vi "LSMcontroller_v66_improvedwfhandling.vi"() -> ()   [LabVIEW 2015] (continued)
                            n1708 = case shown="False" w4683 {
                              frame False {
                                n1709 = disable-structure shown="Disabled" {
                                frame Disabled {
                                n1710 = call "2pparameters.vi"("command"="get") -> ("params out"=w4685:T10)  [unwired: 1 in]
                                n1711 = Unbundle By Name(w4685) -> ("autoshutter"=w4686:bool)
                                n1712 = case shown="True" w4686 {
                                frame False {
                                }
                                frame True {
                                n1713 = call "shuttercontrol.vi"("command"="open") -> ()  [unwired: 1 in, 1 out]
                                }
                                }
                                }
                                frame Enabled {
                                }
                                }
                              }
                              frame True {
                              }
                            }
                          }
                          frame #4 {
                            n1714 = flat-sequence {
                              frame #0 {
                                # "Disabled for conversion to 64 bit"
                                n1715 = disable-structure shown="Disabled" {
                                frame Disabled {
                                n1716 = local read "Measurement"() -> (w4689:T4)
                                n1717 = case shown="\"Lifetime (contour)\"" w4689 {
                                frame "X-Y-t movie", Default {
                                }
                                frame "Lifetime (contour)" {
                                n1718 = call "runLT_img.vi"() -> ()  [unwired: 1 in]
                                }
                                }
                                }
                                frame Enabled {
                                }
                                }
                                n1719 = local write "64bit disabled"(TRUE ("64bit disabled")) -> ()
                              }
                              frame #1 {
                                n1720 = call "runAI_img.vi"() -> ()  [unwired: 12 in]
                                n1721 = call "runCI.vi"() -> ()  [unwired: 12 in]
                                n1722 = call "runDO_img.vi"() -> ()  [unwired: 12 in]
                              }
                              frame #2 {
                                n1723 = call "runAO_img.vi"() -> ()  [unwired: 12 in]
                              }
                            }
                          }
                          frame #5 {
                            # "Disabled for conversion to 64 bit"
                            n1724 = disable-structure shown="Disabled" {
                              disable-tunnel: w4691 -> [w4692 _]
                              frame Disabled {
                                w4695 = u16 0 items=["Stream to disk", "Post process", "real time process"] ("Ring")
                                n1725 = local read "T3R Data processing"() -> (w4694:u16)
                                n1726 = Equal?(x=w4694, y=w4695) -> (x = y?=w4693:bool)
                                n1727 = local read "save\ndata"() -> (w4697:bool)
                                n1728 = local read "Measurement"() -> (w4698:T4)
                                n1729 = And(x=w4697, y=w4693) -> (x .and. y?=w4696:bool)
                                n1730 = case shown="\"Lifetime (contour)\"" w4698 {
                                tunnel: w4692 -> [_ w4702]
                                tunnel: w4696 -> [_ w4700]
                                frame "X-Y-t movie", Default {
                                }
                                frame "Lifetime (contour)" {
                                n1731 = case shown="True" w4700 {
                                selector: w4700 -> [w4703 w4708]
                                tunnel: w4702 -> [_ w4706]
                                tunnel: [path "" ("appended path") w4709] -> w4701
                                tunnel: [w4703 w4708] -> w4699
                                frame False {
                                }
                                frame True {
                                n1732 = local read "filename prefix"() -> (w4707:string)
                                n1733 = local read "data dir"() -> (w4710:path)
                                n1734 = call "generatedatafilename.vi"("timestamp"=w4706, "filename prefix in"=w4707) -> ("full-filename"=w4705:string)
                                n1735 = Concatenate Strings(w4705, ".lvpt3contour" ("string")) -> (w4712:string)
                                n1736 = Build Path(base path=w4710, name or relative path=w4712) -> (appended path=w4709:path)
                                }
                                }
                                n1737 = call "collectLT_res_v1.vi"("stream?"=w4699, "data file"=w4701) -> ()  [unwired: 2 out]
                                }
                                }
                              }
                              frame Enabled {
                              }
                            }
                            n1738 = while {
                              i -> [w4715]
                              stop <- w4713 stop-if-true
                              n1739 = local read "Stop"() -> (w4723:bool)
                              n1740 = local read "Exit"() -> (w4722:bool)
                              n1741 = Increment(x=w4715) -> (x+1=w4714:i32)
                              n1742 = local write "points recorded"(w4714) -> ()
                              n1743 = Or(x=w4723, y=w4722) -> (x .or. y?=w4721:bool)
                              n1744 = case shown="False" w4721 {
                                frame False {
                                n1745 = stacked-sequence {
                                frame #0 {
                                n1746 = call "collectAI_tt_V2.vi"() -> ()  [unwired: 4 in]
                                n1747 = call "collectCI_tt.vi"() -> ("size(s)"=w4730:i32)  [unwired: 3 in]
                                n1748 = local write "scol"(w4730) -> ()
                                }
                                frame #1 {
                                n1749 = local read "Live"() -> (w4731:bool)
                                n1750 = case shown="True" w4731 {
                                frame False {
                                }
                                frame True {
                                n1751 = local read "graph1list"() -> (w4738:u16)
                                n1752 = local read "graph2list"() -> (w4737:u16)
                                n1753 = To Unsigned Word Integer(number=w4738) -> (unsigned 16bit integer=w4736:u16)
                                n1754 = To Unsigned Word Integer(number=w4737) -> (unsigned 16bit integer=w4735:u16)
                                n1755 = call "dattotrace.vi"("graph2list"=w4735, "Current Average"=sgl 1.0, "graph1list"=w4736) -> ("trace2array out"=w4733:sgl[], "trace1array out"=w4744:sgl[])
                                n1756 = local read "bin"() -> (w4745:dbl)
                                n1757 = script code="data=reshape(datain,[bin length(datain)./bin]);\ndataout=mean(data,1);\ndata2=reshape(datain2,[bin length(datain2)./bin]);\ndataout2=mean(data2,1);"("bin"=w4745, "datain"=w4744, "datain2"=w4733) -> ("dataout"=w4743:dbl[], "dataout2"=w4732:dbl[])  [unwired: 1 in, 1 out]
                                n1758 = Array Size(array=w4732) -> (size(s)=w4746:i32)
                                n1759 = Divide(x=w4746, y=2) -> (x/y=w4748:dbl)
                                n1760 = Round To Nearest(number=w4748) -> (nearest integer value=w4750:dbl)
                                n1761 = Array Size(array=w4743) -> (size(s)=w4755:i32)
                                n1762 = Delete From Array(array=w4732, length=w4750, index=0) -> (deleted portion=w4741:dbl[], array with subset deleted=w4742:dbl[])
                                n1763 = Divide(x=w4755, y=2) -> (x/y=w4753:dbl)
                                n1764 = Round To Nearest(number=w4753) -> (nearest integer value=w4751:dbl)
                                n1765 = Delete From Array(array=w4743, length=w4751, index=0) -> (deleted portion=w4740:dbl[], array with subset deleted=w4739:dbl[])
                                n1766 = local write "graph2"(w4739) -> ()
                                n1767 = local write "graph1"(w4740) -> ()
                                n1768 = local write "graph3"(w4741) -> ()
                                n1769 = local write "graph4"(w4742) -> ()
                                }
                                }
                                }
                                frame #2 {
                                n1770 = local read "save\ndata"() -> (w4756:bool)
                                n1771 = case shown="True" w4756 {
                                frame False {
                                }
                                frame True {
                                n1772 = call "savebinaryfiles.vi"() -> ()  [unwired: 1 in]
                                }
                                }
                                }
                                }
                                }
                                frame True {
                                }
                              }
                              n1773 = local read "continuous"() -> (w4718:bool)
                              n1774 = case shown="False" w4718 {
                                tunnel: w4714 -> [w4728 _]
                                tunnel: [w4727 FALSE] -> w4716
                                frame False {
                                n1775 = call "2pparameters.vi"("command"="get") -> ("params out"=w4725:T10)  [unwired: 1 in]
                                n1776 = Unbundle By Name(w4725) -> ("tt_cycles"=w4724:i32)
                                n1777 = Greater Or Equal?(x=w4728, y=w4724) -> (x >= y?=w4727:bool)
                                }
                                frame True {
                                }
                              }
                              n1778 = local read "Stop"() -> (w4720:bool)
                              n1779 = local read "Exit"() -> (w4719:bool)
                              n1780 = Or(x=w4720, y=w4719) -> (x .or. y?=w4717:bool)
                              n1781 = Or(x=w4717, y=w4716) -> (x .or. y?=w4713:bool)
                            }
                            n1782 = local write "64bit disabled"(TRUE ("64bit disabled")) -> ()
                          }
                          frame #6 {
                            # "Disabled for conversion to 64 bit"
                            n1783 = local read "Measurement"() -> (w4759:T4)
                            n1784 = disable-structure shown="Disabled" {
                              disable-tunnel: w4759 -> [w4761 _]
                              disable-tunnel: w4758 -> [w4760 _]
                              frame Disabled {
                                n1785 = case shown="\"Lifetime (contour)\"" w4761 {
                                tunnel: w4760 -> [_ w4762]
                                frame "X-Y-t movie", Default {
                                }
                                frame "Lifetime (contour)" {
                                n1786 = stacked-sequence {
                                tunnel: w4762 -> [_ w4763]
                                frame #0 {
                                n1787 = flat-sequence {
                                frame #0 {
                                n1788 = call "stoperaseLT_img.vi"() -> ()  [unwired: 1 in]
                                }
                                }
                                }
                                frame #1 {
                                w4766 = u16 0 items=["Stream to disk", "Post process", "real time process"] ("Ring")
                                n1789 = local read "T3R Data processing"() -> (w4765:u16)
                                n1790 = local read "save\ndata"() -> (w4768:bool)
                                n1791 = Equal?(x=w4765, y=w4766) -> (x = y?=w4764:bool)
                                n1792 = Not(x=w4764) -> (.not. x?=w4769:bool)
                                n1793 = And(x=w4768, y=w4769) -> (x .and. y?=w4767:bool)
                                n1794 = case shown="True" w4767 {
                                tunnel: w4763 -> [_ w4770]
                                frame False {
                                }
                                frame True {
                                n1795 = local read "filename prefix"() -> (w4771:string)
                                n1796 = local read "data dir"() -> (w4787:path)
                                n1797 = call "2pparameters.vi"("command"="get") -> ("params out"=w4782:T10)  [unwired: 1 in]
                                n1798 = call "generatedatafilename.vi"("timestamp"=w4770, "filename prefix in"=w4771) -> ("full-filename"=w4772:string)
                                n1799 = Unbundle By Name(w4782) -> ("srate"=w4780:sgl, "Pel"=w4779:sgl, "measpoints"=w4777:i32)
                                n1800 = Concatenate Strings(w4772, ".lvpt3contour" ("string")) -> (w4785:string)
                                n1801 = Build Path(base path=w4787, name or relative path=w4785) -> (appended path=w4784:path)
                                n1802 = To Unsigned Long Integer(number=w4780) -> (unsigned 32bit integer=w4781:u32)
                                n1803 = To Unsigned Long Integer(number=w4779) -> (unsigned 32bit integer=w4778:u32)
                                n1804 = To Unsigned Long Integer(number=w4777) -> (unsigned 32bit integer=w4776:u32)
                                n1805 = call "PH-temp-raw.vi"("command"="get") -> ("array out"=w4775:u32[])  [unwired: 1 in]
                                n1806 = Build Array (concatenate)(w4781, w4778, w4776, w4775) -> (w4774:u32[])
                                n1807 = Open/Create/Replace File(file path (use dialog)=w4784, operation (0:open)=T8."replace or create") -> (refnum out=w4791:refnum<file>, error out=w4790:errorcluster)  [unwired: 4 in, 1 out]
                                n1808 = Write to Binary File(file (use dialog)=w4791, data=w4774, error in=w4790, 5:FALSE ("prepend array or string size? (T)")) -> (refnum out=w4788:refnum<file>, error out=w4789:errorcluster)  [unwired: 2 in, 1 out]
                                n1809 = Close File(refnum=w4788, error in=w4789) -> ()  [unwired: 2 out]
                                }
                                }
                                }
                                }
                                }
                                }
                              }
                              frame Enabled {
                              }
                            }
                            n1810 = local write "64bit disabled"(TRUE ("64bit disabled")) -> ()
                          }
                          frame #7 {
                            n1811 = call "reset AO_DO_v3.vi"() -> ()  [unwired: 12 in]
                          }
                          frame #8 {
                            n1812 = stacked-sequence {
                              tunnel: w4807 -> [w4810 _ _ _ _ _]
                              tunnel: w4804 -> [w4809 _ _ _ _ _]
                              tunnel: w4805 -> [w4808 _ _ _ _ _]
                              tunnel: w4806 -> [_ w4859 _ _ _ _]
                              tunnel: w4802 -> [_ w4858 w4913 w5010 _ _]
                              tunnel: w4803 -> [_ w4857 w4912 w5009 _ _]
                              tunnel: w4801 -> [_ _ _ w5008 _ _]
                              tunnel: w4800 -> [_ _ _ w5007 _ _]
                              tunnel: w4799 -> [_ _ w4910 _ _ _]
                              tunnel: w4798 -> [_ _ w4909 _ _ _]
                              tunnel: w4797 -> [_ _ w4907 _ _ _]
                              tunnel: w4796 -> [_ _ w4906 _ _ _]
                              tunnel: w4795 -> [_ _ _ w5005 _ _]
                              tunnel: w4794 -> [_ _ _ w5004 _ _]
                              frame #0 {
                                n1813 = case shown="False" w4810 {
                                tunnel: w4809 -> [_ w4832]
                                tunnel: w4808 -> [_ w4831]
                                frame True {
                                n1814 = stacked-sequence {
                                seq-local: [w4811 _ _] -> [_ w4823 w4828]
                                frame #0 {
                                n1815 = call "configuration.vi"("command"="get") -> ("config out"=w4817:T11)  [unwired: 2 in, 1 out]
                                n1816 = Unbundle By Name(w4817) -> ("Voltage to Xgalvo"=w4814:i32)
                                n1817 = call "2pparameters.vi"("command"="get") -> ("params out"=w4815:T10)  [unwired: 1 in]
                                n1818 = in-place {
                                in-place-border: w4814 -> [w4822]
                                in-place-border: [w4819] -> w4811
                                n1819 = in-place-cluster #31(w4815) -> ("aAO"=w4821:u32[])
                                n1820 = call "remove channel from active arrayv2.vi"("line array in"=w4821, "line to remove"=w4822) -> ("line array out"=w4820:u32[], "index"=w4819:i32)  [unwired: 1 out]
                                n1821 = in-place-cluster #31("aAO"=w4820) -> (w4812:T10)
                                }
                                n1822 = call "2pparameters.vi"("Params in"=w4812, "command"="set") -> ()  [unwired: 1 out]
                                }
                                frame #1 {
                                n1823 = call "waveformparamsv2.vi"("command"="rem AO", "index"=w4823) -> ()  [unwired: 3 in, 3 out]
                                }
                                frame #2 {
                                n1824 = call "waveformsAObuffer.vi"("command"="get") -> ("AO wf out"=w4829:waveform(dbl)[])  [unwired: 1 in]
                                n1825 = Delete From Array(array=w4829, length=1, index=w4828) -> (array with subset deleted=w4825:waveform(dbl)[])  [unwired: 1 out]
                                n1826 = call "waveformsAObuffer.vi"("AO wf in"=w4825, "command"="set") -> ()  [unwired: 1 out]
                                }
                                }
                                }
                                frame False {
                                n1827 = stacked-sequence {
                                seq-local: [w4833 _ _] -> [_ w4841 w4852]
                                tunnel: w4832 -> [_ w4840 _]
                                tunnel: w4831 -> [_ _ w4851]
                                frame #0 {
                                n1828 = call "configuration.vi"("command"="get") -> ("config out"=w4838:T11)  [unwired: 2 in, 1 out]
                                n1829 = Unbundle By Name(w4838) -> ("Voltage to Xgalvo"=w4834:i32)
                                n1830 = call "2pparameters.vi"("command"="get") -> ("params out"=w4837:T10)  [unwired: 1 in]
                                n1831 = Unbundle By Name(w4837) -> ("aAO"=w4835:u32[])
                                n1832 = Search 1D Array(1D array=w4835, element=w4834) -> (index of element=w4833:i32)  [unwired: 1 in]
                                }
                                frame #1 {
                                n1833 = call "waveformparamsv2.vi"("command"="get") -> ("Params out"=w4844:T14)  [unwired: 4 in, 2 out]
                                n1834 = in-place {
                                in-place-border: w4841 -> [w4848]
                                in-place-border: w4840 -> [w4847]
                                n1835 = in-place-cluster #32(w4844) -> ("AO parameters"=w4849:T15)
                                n1836 = in-place {
                                in-place-border: w4847 -> [w4850]
                                n1837 = in-place-array #33(w4849, w4848) -> ()  [unwired: 1 out]
                                n1838 = in-place-array #33(w4850) -> (w4846:T15)  [unwired: 1 out]
                                }
                                n1839 = in-place-cluster #32("AO parameters"=w4846) -> (w4842:T14)
                                }
                                n1840 = call "waveformparamsv2.vi"("command"="set", "Params in"=w4842) -> ()  [unwired: 3 in, 3 out]
                                }
                                frame #2 {
                                n1841 = call "waveformsAObuffer.vi"("command"="get") -> ("AO wf out"=w4855:waveform(dbl)[])  [unwired: 1 in]
                                n1842 = Replace Array Subset(array=w4855, new element=w4851, index=w4852) -> (w4853:waveform(dbl)[])
                                n1843 = call "waveformsAObuffer.vi"("AO wf in"=w4853, "command"="set") -> ()  [unwired: 1 out]
                                }
                                }
                                }
                                }
                              }
                              frame #1 {
                                n1844 = case shown="False" w4859 {
                                tunnel: w4858 -> [_ w4881]
                                tunnel: w4857 -> [_ w4880]
                                frame True {
                                n1845 = stacked-sequence {
                                seq-local: [w4860 _ _] -> [_ w4872 w4877]
                                frame #0 {
                                n1846 = call "configuration.vi"("command"="get") -> ("config out"=w4866:T11)  [unwired: 2 in, 1 out]
                                n1847 = Unbundle By Name(w4866) -> ("Voltage to Ygalvo"=w4863:i32)
                                n1848 = call "2pparameters.vi"("command"="get") -> ("params out"=w4864:T10)  [unwired: 1 in]
                                n1849 = in-place {
                                in-place-border: w4863 -> [w4871]
                                in-place-border: [w4868] -> w4860
                                n1850 = in-place-cluster #34(w4864) -> ("aAO"=w4870:u32[])
                                n1851 = call "remove channel from active arrayv2.vi"("line array in"=w4870, "line to remove"=w4871) -> ("line array out"=w4869:u32[], "index"=w4868:i32)  [unwired: 1 out]
                                n1852 = in-place-cluster #34("aAO"=w4869) -> (w4861:T10)
                                }
                                n1853 = call "2pparameters.vi"("Params in"=w4861, "command"="set") -> ()  [unwired: 1 out]
                                }
                                frame #1 {
                                n1854 = call "waveformparamsv2.vi"("command"="rem AO", "index"=w4872) -> ()  [unwired: 3 in, 3 out]
                                }
                                frame #2 {
                                n1855 = call "waveformsAObuffer.vi"("command"="get") -> ("AO wf out"=w4878:waveform(dbl)[])  [unwired: 1 in]
                                n1856 = Delete From Array(array=w4878, length=1, index=w4877) -> (array with subset deleted=w4874:waveform(dbl)[])  [unwired: 1 out]
                                n1857 = call "waveformsAObuffer.vi"("AO wf in"=w4874, "command"="set") -> ()  [unwired: 1 out]
                                }
                                }
                                }
                                frame False {
                                n1858 = stacked-sequence {
                                seq-local: [w4882 _ _] -> [_ w4890 w4901]
                                tunnel: w4881 -> [_ w4889 _]
                                tunnel: w4880 -> [_ _ w4900]
                                frame #0 {
                                n1859 = call "configuration.vi"("command"="get") -> ("config out"=w4887:T11)  [unwired: 2 in, 1 out]
                                n1860 = Unbundle By Name(w4887) -> ("Voltage to Ygalvo"=w4883:i32)
                                n1861 = call "2pparameters.vi"("command"="get") -> ("params out"=w4886:T10)  [unwired: 1 in]
                                n1862 = Unbundle By Name(w4886) -> ("aAO"=w4884:u32[])
                                n1863 = Search 1D Array(1D array=w4884, element=w4883) -> (index of element=w4882:i32)  [unwired: 1 in]
                                }
                                frame #1 {
                                n1864 = call "waveformparamsv2.vi"("command"="get") -> ("Params out"=w4893:T14)  [unwired: 4 in, 2 out]
                                n1865 = in-place {
                                in-place-border: w4890 -> [w4897]
                                in-place-border: w4889 -> [w4896]
                                n1866 = in-place-cluster #35(w4893) -> ("AO parameters"=w4898:T15)
                                n1867 = in-place {
                                in-place-border: w4896 -> [w4899]
                                n1868 = in-place-array #36(w4898, w4897) -> ()  [unwired: 1 out]
                                n1869 = in-place-array #36(w4899) -> (w4895:T15)  [unwired: 1 out]
                                }
                                n1870 = in-place-cluster #35("AO parameters"=w4895) -> (w4891:T14)
                                }
                                n1871 = call "waveformparamsv2.vi"("command"="set", "Params in"=w4891) -> ()  [unwired: 3 in, 3 out]
                                }
                                frame #2 {
                                n1872 = call "waveformsAObuffer.vi"("command"="get") -> ("AO wf out"=w4904:waveform(dbl)[])  [unwired: 1 in]
                                n1873 = Replace Array Subset(array=w4904, new element=w4900, index=w4901) -> (w4902:waveform(dbl)[])
                                n1874 = call "waveformsAObuffer.vi"("AO wf in"=w4902, "command"="set") -> ()  [unwired: 1 out]
                                }
                                }
                                }
                                }
                              }
                              frame #2 {
                                n1875 = Build Array(w4910, w4909) -> (w4911:bool[])
                                n1876 = Boolean Array To Number(Boolean array=w4911) -> (number=w4908:u32)
                                n1877 = case shown="2" w4908 {
                                tunnel: w4913 -> [_ _ w4956]
                                tunnel: w4912 -> [_ _ w4955]
                                tunnel: w4907 -> [_ w4935 w4954]
                                tunnel: w4906 -> [_ w4934 w4953]
                                frame 1, Default {
                                n1878 = stacked-sequence {
                                seq-local: [w4914 _ _] -> [_ w4926 w4931]
                                frame #0 {
                                n1879 = call "configuration.vi"("command"="get") -> ("config out"=w4920:T11)  [unwired: 2 in, 1 out]
                                n1880 = Unbundle By Name(w4920) -> ("2P shutter"=w4917:i32)
                                n1881 = call "2pparameters.vi"("command"="get") -> ("params out"=w4918:T10)  [unwired: 1 in]
                                n1882 = in-place {
                                in-place-border: w4917 -> [w4925]
                                in-place-border: [w4922] -> w4914
                                n1883 = in-place-cluster #37(w4918) -> ("aDO"=w4924:u32[])
                                n1884 = call "remove channel from active arrayv2.vi"("line array in"=w4924, "line to remove"=w4925) -> ("line array out"=w4923:u32[], "index"=w4922:i32)  [unwired: 1 out]
                                n1885 = in-place-cluster #37("aDO"=w4923) -> (w4915:T10)
                                }
                                n1886 = call "2pparameters.vi"("Params in"=w4915, "command"="set") -> ()  [unwired: 1 out]
                                }
                                frame #1 {
                                n1887 = call "waveformparamsv2.vi"("command"="rem DO", "index"=w4926) -> ()  [unwired: 3 in, 3 out]
                                }
                                frame #2 {
                                n1888 = call "waveformsDObuffer.vi"("command"="get") -> ("DO wf out"=w4932:digitalwaveform[])  [unwired: 1 in]
                                n1889 = Delete From Array(array=w4932, length=1, index=w4931) -> (array with subset deleted=w4928:digitalwaveform[])  [unwired: 1 out]
                                n1890 = call "waveformsDObuffer.vi"("DO wf in"=w4928, "command"="set") -> ()  [unwired: 1 out]
                                }
                                }
                                }
                                frame 2 {
                                n1891 = stacked-sequence {
                                tunnel: w4935 -> [_ w4946 _]
                                tunnel: w4934 -> [_ _ w4948]
                                frame #0 {
                                n1892 = call "configuration.vi"("command"="get") -> ("config out"=w4937:T11)  [unwired: 2 in, 1 out]
                                n1893 = call "2pparameters.vi"("command"="get") -> ("params out"=w4941:T10)  [unwired: 1 in]
                                n1894 = Unbundle By Name(w4937) -> ("2P shutter"=w4936:i32)
                                n1895 = in-place {
                                in-place-border: w4936 -> [w4945]
                                n1896 = in-place-cluster #38(w4941) -> ("aDO"=w4944:u32[])
                                n1897 = call "add channel to active arrayv2.vi"("line array in"=w4944, "line to add"=w4945) -> ("line array out"=w4943:u32[])  [unwired: 2 out]
                                n1898 = in-place-cluster #38("aDO"=w4943) -> (w4939:T10)
                                }
                                n1899 = call "2pparameters.vi"("Params in"=w4939, "command"="set") -> ()  [unwired: 1 out]
                                }
                                frame #1 {
                                n1900 = call "waveformparamsv2.vi"("command"="add DO", "add DO"=w4946) -> ()  [unwired: 3 in, 3 out]
                                }
                                frame #2 {
                                n1901 = call "waveformsDObuffer.vi"("command"="get") -> ("DO wf out"=w4951:digitalwaveform[])  [unwired: 1 in]
                                n1902 = Build Array (concatenate)(w4951, w4948) -> (w4950:digitalwaveform[])
                                n1903 = call "waveformsDObuffer.vi"("DO wf in"=w4950, "command"="set") -> ()  [unwired: 1 out]
                                }
                                }
                                }
                                frame 0 {
                                n1904 = stacked-sequence {
                                seq-local: [w4957 _ _] -> [_ w4965 w4987]
                                tunnel: w4956 -> [_ _ _]
                                tunnel: w4955 -> [_ _ _]
                                tunnel: w4954 -> [_ w4964 _]
                                tunnel: w4953 -> [_ _ w4986]
                                frame #0 {
                                n1905 = call "configuration.vi"("command"="get") -> ("config out"=w4962:T11)  [unwired: 2 in, 1 out]
                                n1906 = call "2pparameters.vi"("command"="get") -> ("params out"=w4961:T10)  [unwired: 1 in]
                                n1907 = Unbundle By Name(w4962) -> ("2P shutter"=w4958:i32)
                                n1908 = Unbundle By Name(w4961) -> ("aDO"=w4959:u32[])
                                n1909 = Search 1D Array(1D array=w4959, element=w4958) -> (index of element=w4957:i32)  [unwired: 1 in]
                                }
                                frame #1 {
                                n1910 = call "2pparameters.vi"("command"="get") -> ("params out"=w4968:T10)  [unwired: 1 in]
                                n1911 = Unbundle By Name(w4968) -> ("wavdet"=w4966:bool, "autoshutter"=w4967:bool)
                                n1912 = case shown="True" w4967 {
                                tunnel: w4965 -> [_ w4972]
                                tunnel: w4966 -> [_ w4971]
                                tunnel: w4964 -> [_ w4970]
                                frame False {
                                }
                                frame True {
                                n1913 = case shown="False" w4971 {
                                tunnel: w4972 -> [w4976 _]
                                tunnel: w4970 -> [w4973 _]
                                frame False {
                                n1914 = Index Array(array=w4973, index=0) -> (element=w4974:T18)
                                n1915 = call "waveformparamsv2.vi"("command"="get") -> ("Params out"=w4979:T14)  [unwired: 4 in, 2 out]
                                n1916 = in-place {
                                in-place-border: w4976 -> [w4983]
                                in-place-border: w4974 -> [w4981]
                                n1917 = in-place-cluster #39(w4979) -> ("DO parameters"=w4984:T17)
                                n1918 = in-place {
                                in-place-border: w4981 -> [w4985]
                                n1919 = in-place-array #40(w4984, w4983) -> ()  [unwired: 1 out]
                                n1920 = in-place-array #40(w4985) -> (w4982:T17)  [unwired: 1 out]
                                }
                                n1921 = in-place-cluster #39("DO parameters"=w4982) -> (w4977:T14)
                                }
                                n1922 = call "waveformparamsv2.vi"("command"="set", "Params in"=w4977) -> ()  [unwired: 3 in, 3 out]
                                }
                                frame True {
                                }
                                }
                                }
                                }
                                }
                                frame #2 {
                                n1923 = call "2pparameters.vi"("command"="get") -> ("params out"=w4990:T10)  [unwired: 1 in]
                                n1924 = Unbundle By Name(w4990) -> ("wavdet"=w4988:bool, "autoshutter"=w4989:bool)
                                n1925 = case shown="True" w4989 {
                                tunnel: w4987 -> [_ w4994]
                                tunnel: w4988 -> [_ w4993]
                                tunnel: w4986 -> [_ w4992]
                                frame False {
                                }
                                frame True {
                                n1926 = case shown="False" w4993 {
                                tunnel: w4994 -> [w4998 _]
                                tunnel: w4992 -> [w4996 _]
                                frame False {
                                n1927 = Index Array(array=w4996, index=0) -> (element=w4995:digitalwaveform)
                                n1928 = call "waveformsDObuffer.vi"("command"="get") -> ("DO wf out"=w5000:digitalwaveform[])  [unwired: 1 in]
                                n1929 = Replace Array Subset(array=w5000, new element=w4995, index=w4998) -> (w5002:digitalwaveform[])
                                n1930 = call "waveformsDObuffer.vi"("DO wf in"=w5002, "command"="set") -> ()  [unwired: 1 out]
                                }
                                frame True {
                                }
                                }
                                }
                                }
                                }
                                }
                                }
                                }
                              }
                              frame #3 {
                                n1931 = Build Array(w5005, w5004) -> (w5006:bool[])
                                n1932 = Boolean Array To Number(Boolean array=w5006) -> (number=w5003:u32)
                                n1933 = case shown="2" w5003 {
                                tunnel: w5010 -> [_ _ w5053]
                                tunnel: w5009 -> [_ _ w5052]
                                tunnel: w5008 -> [_ w5032 w5050]
                                tunnel: w5007 -> [_ w5031 w5051]
                                frame 1, Default {
                                n1934 = stacked-sequence {
                                seq-local: [w5011 _ _] -> [_ w5023 w5028]
                                frame #0 {
                                n1935 = call "configuration.vi"("command"="get") -> ("config out"=w5017:T11)  [unwired: 2 in, 1 out]
                                n1936 = Unbundle By Name(w5017) -> ("LT timestamp"=w5014:u32)
                                n1937 = call "2pparameters.vi"("command"="get") -> ("params out"=w5015:T10)  [unwired: 1 in]
                                n1938 = in-place {
                                in-place-border: w5014 -> [w5022]
                                in-place-border: [w5019] -> w5011
                                n1939 = in-place-cluster #41(w5015) -> ("aDO"=w5021:u32[])
                                n1940 = call "remove channel from active arrayv2.vi"("line array in"=w5021, "line to remove"=w5022) -> ("line array out"=w5020:u32[], "index"=w5019:i32)  [unwired: 1 out]
                                n1941 = in-place-cluster #41("aDO"=w5020) -> (w5012:T10)
                                }
                                n1942 = call "2pparameters.vi"("Params in"=w5012, "command"="set") -> ()  [unwired: 1 out]
                                }
                                frame #1 {
                                n1943 = call "waveformparamsv2.vi"("command"="rem DO", "index"=w5023) -> ()  [unwired: 3 in, 3 out]
                                }
                                frame #2 {
                                n1944 = call "waveformsDObuffer.vi"("command"="get") -> ("DO wf out"=w5029:digitalwaveform[])  [unwired: 1 in]
                                n1945 = Delete From Array(array=w5029, length=1, index=w5028) -> (array with subset deleted=w5025:digitalwaveform[])  [unwired: 1 out]
                                n1946 = call "waveformsDObuffer.vi"("DO wf in"=w5025, "command"="set") -> ()  [unwired: 1 out]
                                }
                                }
                                }
                                frame 2 {
                                n1947 = stacked-sequence {
                                tunnel: w5032 -> [_ _ w5045]
                                tunnel: w5031 -> [_ w5043 _]
                                frame #0 {
                                n1948 = call "configuration.vi"("command"="get") -> ("config out"=w5034:T11)  [unwired: 2 in, 1 out]
                                n1949 = Unbundle By Name(w5034) -> ("LT timestamp"=w5033:u32)
                                n1950 = call "2pparameters.vi"("command"="get") -> ("params out"=w5038:T10)  [unwired: 1 in]
                                n1951 = in-place {
                                in-place-border: w5033 -> [w5042]
                                n1952 = in-place-cluster #42(w5038) -> ("aDO"=w5041:u32[])
                                n1953 = call "add channel to active arrayv2.vi"("line array in"=w5041, "line to add"=w5042) -> ("line array out"=w5040:u32[])  [unwired: 2 out]
                                n1954 = in-place-cluster #42("aDO"=w5040) -> (w5036:T10)
                                }
                                n1955 = call "2pparameters.vi"("Params in"=w5036, "command"="set") -> ()  [unwired: 1 out]
                                }
                                frame #1 {
                                n1956 = call "waveformparamsv2.vi"("command"="add DO", "add DO"=w5043) -> ()  [unwired: 3 in, 3 out]
                                }
                                frame #2 {
                                n1957 = call "waveformsDObuffer.vi"("command"="get") -> ("DO wf out"=w5048:digitalwaveform[])  [unwired: 1 in]
                                n1958 = Build Array (concatenate)(w5048, w5045) -> (w5047:digitalwaveform[])
                                n1959 = call "waveformsDObuffer.vi"("DO wf in"=w5047, "command"="set") -> ()  [unwired: 1 out]
                                }
                                }
                                }
                                frame 0 {
                                n1960 = stacked-sequence {
                                seq-local: [w5054 _ _] -> [_ w5064 w5081]
                                tunnel: w5053 -> [_ _ _]
                                tunnel: w5052 -> [_ _ _]
                                tunnel: w5051 -> [_ w5061 _]
                                tunnel: w5050 -> [_ _ w5080]
                                frame #0 {
                                n1961 = call "configuration.vi"("command"="get") -> ("config out"=w5059:T11)  [unwired: 2 in, 1 out]
                                n1962 = Unbundle By Name(w5059) -> ("LT timestamp"=w5055:u32)
                                n1963 = call "2pparameters.vi"("command"="get") -> ("params out"=w5058:T10)  [unwired: 1 in]
                                n1964 = Unbundle By Name(w5058) -> ("aDO"=w5056:u32[])
                                n1965 = Search 1D Array(1D array=w5056, element=w5055) -> (index of element=w5054:i32)  [unwired: 1 in]
                                }
                                frame #1 {
                                n1966 = local read "Measurement"() -> (w5063:T4)
                                n1967 = To Unsigned Long Integer(number=w5063) -> (unsigned 32bit integer=w5062:u32)
                                n1968 = case shown="5..7" w5062 {
                                tunnel: w5064 -> [_ w5068]
                                tunnel: w5061 -> [_ w5065]
                                frame 0..4, Default {
                                }
                                frame 5..7 {
                                n1969 = Index Array(array=w5065, index=0) -> (element=w5066:T18)
                                n1970 = call "waveformparamsv2.vi"("command"="get") -> ("Params out"=w5071:T14)  [unwired: 4 in, 2 out]
                                n1971 = in-place {
                                in-place-border: w5068 -> [w5075]
                                in-place-border: w5066 -> [w5073]
                                n1972 = in-place-cluster #43(w5071) -> ("DO parameters"=w5076:T17)
                                n1973 = in-place {
                                in-place-border: w5073 -> [w5077]
                                n1974 = in-place-array #44(w5076, w5075) -> ()  [unwired: 1 out]
                                n1975 = in-place-array #44(w5077) -> (w5074:T17)  [unwired: 1 out]
                                }
                                n1976 = in-place-cluster #43("DO parameters"=w5074) -> (w5069:T14)
                                }
                                n1977 = call "waveformparamsv2.vi"("command"="set", "Params in"=w5069) -> ()  [unwired: 3 in, 3 out]
                                }
                                }
                                }
                                frame #2 {
                                n1978 = local read "Measurement"() -> (w5079:T4)
                                n1979 = To Unsigned Long Integer(number=w5079) -> (unsigned 32bit integer=w5078:u32)
                                n1980 = case shown="5..7" w5078 {
                                tunnel: w5081 -> [_ w5085]
                                tunnel: w5080 -> [_ w5083]
                                frame 0..4, Default {
                                }
                                frame 5..7 {
                                n1981 = Index Array(array=w5083, index=0) -> (element=w5082:digitalwaveform)
                                n1982 = call "waveformsDObuffer.vi"("command"="get") -> ("DO wf out"=w5087:digitalwaveform[])  [unwired: 1 in]
                                n1983 = Replace Array Subset(array=w5087, new element=w5082, index=w5085) -> (w5089:digitalwaveform[])
                                n1984 = call "waveformsDObuffer.vi"("DO wf in"=w5089, "command"="set") -> ()  [unwired: 1 out]
                                }
                                }
                                }
                                }
                                }
                                }
                              }
                              frame #4 {
                                n1985 = call "Used AO lines.vi"() -> ("used AO names"=w5092:string[], "used AO lines"=w5090:tag[])  [unwired: 2 in]
                                n1986 = control-ref of="Analog Lines Plot"() -> (w5091:refnum<vi>)
                                n1987 = control-ref of="Digital Lines Plot"() -> (w5093:refnum<vi>)
                                n1988 = call "Used DO lines.vi"() -> ("used DO names"=w5094:string[], "used DO lines"=w5095:tag[])  [unwired: 2 in]
                                n1989 = local write "Analog Used Lines"(w5090) -> ()
                                n1990 = local write "Analog Used Names"(w5092) -> ()
                                n1991 = local write "Digital Used Lines"(w5095) -> ()
                                n1992 = local write "Digital Used Names"(w5094) -> ()
                                n1993 = call "prepDOWaveplot.vi"("DigitalGraph in"=w5093, "used DO names"=w5094) -> ()  [unwired: 1 in]
                                n1994 = call "prepAOWaveplot.vi"("WaveformGraph in"=w5091, "Analog Used Names"=w5092) -> ()  [unwired: 1 in]
                              }
                              frame #5 {
                                n1995 = local read "Meastab"() -> (w5110:enum32{"X-Y Image", "Linescan", "Timetrace"})
                                n1996 = property on="refwf" class="Ring (strict)"() -> ("RingText.Text"=w5107:string)  [unwired: 2 in, 2 out]
                                n1997 = case shown="\"Timetrace\"" w5110 {
                                tunnel: [w5112 w5113] -> w5111
                                frame "X-Y Image", Default {
                                n1998 = local read "Sampling rate"() -> (w5112:dbl)
                                }
                                frame "Timetrace" {
                                n1999 = local read "srateAODOtt"() -> (w5113:dbl)
                                }
                                }
                                n2000 = call "waveformsAObuffer.vi"("command"="get") -> ("AO wf out"=w5098:waveform(dbl)[])  [unwired: 1 in]
                                n2001 = local read "wavdet"() -> (w5108:bool)
                                n2002 = call "waveformsDObuffer.vi"("command"="get") -> ("DO wf out"=w5102:digitalwaveform[])  [unwired: 1 in]
                                n2003 = call "correctwaveformsizetemp.vi"("new sampling frequency (Hz)"=w5111, "start"=FALSE, "reference waveforms to"=w5107, "Analog waveforms in"=w5098, "stop"=TRUE, "Digital waveforms in"=w5102) -> ("analog wf out"=w5104:waveform(dbl)[], "Digital wf out"=w5106:digitalwaveform[], "measpoints"=w5109:i32)
                                n2004 = local write "Analog Lines Plot"(w5104) -> ()
                                n2005 = call "GetNumCamFramesv2.vi"("Digital Waveform Graph"=w5106) -> ("Numeric"=w5105:i32)  [unwired: 10 in]
                                n2006 = local write "Digital Lines Plot"(w5106) -> ()
                                n2007 = call "waveformsDObuffer.vi"("DO wf in"=w5106, "command"="set") -> ()  [unwired: 1 out]
                                n2008 = call "waveformsAObuffer.vi"("AO wf in"=w5104, "command"="set") -> ()  [unwired: 1 out]
                                n2009 = local write "Total Camera Frames"(w5105) -> ()
                                n2010 = case shown="True" w5108 {
                                tunnel: w5109 -> [_ w5114]
                                frame False {
                                }
                                frame True {
                                n2011 = local write "# of frames"(w5114) -> ()
                                }
                                }
                              }
                            }
                            n2012 = call "stoperaseCI.vi"() -> ()  [unwired: 12 in]
                            n2013 = call "stoperaseDO_img.vi"() -> ()  [unwired: 12 in]
                            n2014 = call "stoperaseAO_img.vi"() -> ()  [unwired: 12 in]
                            n2015 = call "stoperaseAI_img.vi"() -> ()  [unwired: 12 in]
                          }
                          frame #9 {
                            w5124 = FALSE ("Value (Signaling)")
                            n2016 = local read "save\ndata"() -> (w5119:bool)
                            n2017 = case shown="True" w5119 {
                              tunnel: w5118 -> [_ w5131]
                              frame False {
                              }
                              frame True {
                                n2018 = call "closebinaryfiles.vi"() -> ()  [unwired: 12 in]
                                n2019 = local read "filename prefix"() -> (w5133:string)
                                n2020 = local read "data dir"() -> (w5132:path)
                                n2021 = call "saveparams.vi"("timestamp"=w5131, "filename prefix in"=w5133, "data dir in"=w5132) -> ()  [unwired: 1 in]
                              }
                            }
                            n2022 = call "2pparameters.vi"("command"="get") -> ("params out"=w5115:T10)  [unwired: 1 in]
                            n2023 = Unbundle By Name(w5115) -> ("auto OD"=w5116:bool)
                            n2024 = case shown="True" w5116 {
                              frame False {
                              }
                              frame True {
                                n2025 = call "configuration.vi"("command"="get") -> ("config out"=w5127:T11)  [unwired: 2 in, 1 out]
                                n2026 = call "2pparameters.vi"("command"="get") -> ("params out"=w5130:T10)  [unwired: 1 in]
                                n2027 = Unbundle By Name(w5127) -> ("contour OD"=w5125:u16)
                                n2028 = Unbundle By Name(w5130) -> ("ODfilt"=w5126:u16)
                                n2029 = call "filterwheelcontrol_nothorlabslib.vi"("Current OD filt"=w5125, "New ODfilt"=w5126) -> ()  [unwired: 1 in]
                              }
                            }
                            n2030 = property on="Start" class="Bool (strict)"("Val(Sgnl)"=w5124) -> ()  [unwired: 2 in, 2 out]
                            n2031 = property on="Start" class="Bool (strict)"("Visible"=TRUE, "DisabledEnum"=T7."Enabled" ("Disabled")) -> ()  [unwired: 2 in, 2 out]
                            n2032 = property on="Stop" class="Bool (strict)"("Val(Sgnl)"=w5124) -> ()  [unwired: 2 in, 2 out]
                            n2033 = property on="Stop" class="Bool (strict)"("Visible"=FALSE, "DisabledEnum"=T7."Disabled" ("Disabled")) -> ()  [unwired: 2 in, 2 out]
                          }
                          frame #10 {
                            w5136 = T21 2 items=["no dialog", "OK message", "continue or stop message", "OK message + warnings", "continue/stop + warnings"] ("type of dialog (OK msg:1)")
                            n2034 = call "displayerrors.vi"() -> ("error IO"=w5137:errorcluster)
                            n2035 = call <vilib>:"General Error Handler.vi"("type of dialog (OK msg:1)"=w5136, "error in (no error)"=w5137) -> ("error out"=w5135:errorcluster)  [unwired: 9 in, 4 out]
                            n2036 = call <vilib>:"Clear Errors.vi"("error in (no error)"=w5135) -> ("error out"=w5134:errorcluster)  [unwired: 5 in, 1 out]
                            n2037 = call "seterrors.vi"("error IO"=w5134) -> ()
                          }
                        }
                      }
                    }
                  }
                  frame "Lifetime (point)" {
                    # "Disabled for conversion to 64 bit"
                    n2038 = disable-structure shown="Disabled" {
                      frame Disabled {
                        n2039 = stacked-sequence {
                          frame #0 {
                            w5148 = 12.5 ("x")
                            # "get from syncrate"
                            n2040 = local read "Bin size"() -> (w5142:T6)
                            n2041 = local read "Vx-ref"() -> (w5154:dbl)
                            n2042 = local read "Vy-ref"() -> (w5155:dbl)
                            n2043 = call "2pparameters.vi"("command"="get") -> ("params out"=w5140:T10)  [unwired: 1 in]
                            n2044 = Scale By Power Of 2(n=w5142, x=1.0 ("Y Scale.Range:Minimum")) -> (x*2^n=w5151:dbl)
                            n2045 = call "setposition.vi"("Vy"=w5155, "Vx"=w5154) -> ()  [unwired: 1 in]
                            n2046 = Unbundle By Name(w5140) -> ("autoshutter"=w5141:bool)
                            n2047 = Multiply(x=3000.0 ("Y Scale.Range:Minimum"), y=w5151) -> (x*y=w5149:dbl)
                            n2048 = Compound Arithmetic op=MULTIPLY(w5148, invert 3200.0 ("X Scale.Offset and Multiplier:Multiplier"), w5151) -> (w5150:dbl)
                            n2049 = case shown="True" w5141 {
                              frame False {
                              }
                              frame True {
                                n2050 = call "shuttercontrol.vi"("command"="open") -> ()  [unwired: 1 in, 1 out]
                              }
                            }
                            n2051 = call "lifetimeparameters.vi"("command"="get") -> ("Params out"=w5146:T19)  [unwired: 1 in]
                            n2052 = property on="Histogram" class="WFGraph (strict)"("XScale.Maximum"=w5148, "XScale.Minimum"=0.0 ("X Scale.Range:Minimum"), "YScale.Maximum"=w5149, "YScale.Minimum"=0.1 ("Y Scale.Range:Minimum"), "XScale.Multiplier"=w5150) -> ()  [unwired: 2 in, 2 out]
                            n2053 = Bundle By Name(cluster=w5146, "Bin size"=w5142) -> (w5147:T19)
                            n2054 = call "lifetimeparameters.vi"("Params in"=w5147, "command"="set") -> ()  [unwired: 1 out]
                            n2055 = property on="Histogram 2" class="WFGraph (strict)"("YScale.Maximum"=w5149, "XScale.Multiplier"=w5150, "XScale.Maximum"=w5148) -> ()  [unwired: 2 in, 2 out]
                            n2056 = call "2pparameters.vi"("command"="get") -> ("params out"=w5162:T10)  [unwired: 1 in]
                            n2057 = Bundle By Name(cluster=w5162, "type"="Lifetime (point)") -> (w5160:T10)
                            n2058 = property on="Stop" class="Bool (strict)"("Visible"=TRUE, "DisabledEnum"=T7."Enabled" ("Disabled")) -> ()  [unwired: 2 in, 2 out]
                            n2059 = property on="Start" class="Bool (strict)"("Visible"=FALSE, "DisabledEnum"=T7."Disabled and Grayed Out" ("Disabled")) -> ()  [unwired: 2 in, 2 out]
                            n2060 = call "2pparameters.vi"("Params in"=w5160, "command"="set") -> ()  [unwired: 1 out]
                          }
                          frame #1 {
                            n2061 = call "setup.vi"() -> ()  [unwired: 1 in]
                          }
                          frame #2 {
                            # "main loop"
                            n2062 = call "lifetimeparameters.vi"("command"="get") -> ("Params out"=w5172:T19)  [unwired: 1 in]
                            n2063 = Unbundle By Name(w5172) -> ("devidx"=w5170:i32)
                            n2064 = for {
                              N: 10000 -> [_]
                              tunnel: [w5173] -> w5168 mode=indexing
                              i -> [w5173]
                            }
                            n2065 = while {
                              tunnel: w5170 -> [w5177]
                              tunnel: w5168 -> [w5174]
                              i -> [w5175]
                              stop <- w5179 stop-if-true
                              n2066 = Increment(x=w5175) -> (x+1=w5176:i32)
                              n2067 = dll-call lib="phlib.dll" fn="_PH_GetCountRate@8" label="PH_GetCountRate"("devidx"=w5177, "channel"=0) -> (w5178:i32)  [unwired: 5 in, 2 out]
                              "SyncRate" <- w5178
                              n2068 = stacked-sequence {
                                seq-local: [_ _ w5186 _ _] -> [_ _ _ w5199 _]
                                seq-local: [_ _ w5185 _ _] -> [_ _ _ w5198 _]
                                seq-local: [_ w5183 _ _ _] -> [_ _ w5187 _ _]
                                tunnel: w5178 -> [_ _ _ w5206 _]
                                tunnel: w5174 -> [_ _ _ w5196 _]
                                frame #0 {
                                n2069 = call "start_binned.vi"() -> ()  [unwired: 1 in]
                                }
                                frame #1 {
                                n2070 = call "get-histogram.vi"() -> ("IntegralCount"=→"Integral count":u32, "Histogram"=w5183:u32[])
                                "Histogram" <- w5183
                                }
                                frame #2 {
                                n2071 = Search 1D Array(1D array=w5187, element=u32 0) -> (index of element=w5185:i32)  [unwired: 1 in]
                                n2072 = Multiply(x=w5185, y=0.99) -> (x*y=w5191:dbl)
                                n2073 = Array Subset(array=w5187, index=0, length=w5191) -> (w5194:u32[])
                                n2074 = Array Max & Min(array=w5194) -> (max index (indices)=w5188:i32)  [unwired: 3 out]
                                n2075 = Split 1D Array(array=w5194, index=w5188) -> (second subarray=w5190:u32[])  [unwired: 1 out]
                                n2076 = Array Max & Min(array=w5190) -> (min index (indices)=w5189:i32)  [unwired: 3 out]
                                n2077 = Split 1D Array(array=w5190, index=w5189) -> (first subarray=w5186:u32[])  [unwired: 1 out]
                                "Histogram 2" <- w5186
                                }
                                frame #3 {
                                n2078 = Array Size(array=w5199) -> (size(s)=w5201:i32)
                                n2079 = Array Subset(array=w5196, index=0, length=w5201) -> (w5200:i32[])
                                n2080 = Compound Arithmetic op=MULTIPLY(1000000000.0 ("value"), invert w5206, invert w5198, w5200) -> (w5197:dbl[])
                                n2081 = call <vilib>:"Exponential Fit.vi"("Y"=w5199, "X"=w5197) -> ("damping"=w5203:dbl)  [unwired: 8 in, 5 out]
                                n2082 = Divide(x=-1.0 ("y"), y=w5203) -> (x/y=→"Lifetime (ns)":dbl)
                                }
                                frame #4 {
                                n2083 = local read "downright"() -> (w5213:bool)
                                n2084 = local read "downleft"() -> (w5215:bool)
                                n2085 = local read "upright"() -> (w5211:bool)
                                n2086 = local read "upleft"() -> (w5209:bool)
                                n2087 = local read "down"() -> (w5214:bool)
                                n2088 = local read "right"() -> (w5212:bool)
                                n2089 = local read "left"() -> (w5216:bool)
                                n2090 = local read "up"() -> (w5210:bool)
                                n2091 = Compound Arithmetic op=OR(w5209, w5210, w5211, w5212, w5213, w5214, w5215, w5216) -> (w5208:bool)
                                n2092 = case shown="True" w5208 {
                                frame False {
                                }
                                frame True {
                                n2093 = stacked-sequence {
                                frame #0 {
                                n2094 = local read "downright"() -> (w5218:bool)
                                n2095 = local read "downleft"() -> (w5220:bool)
                                n2096 = local read "BigSmall"() -> (w5217:bool)
                                n2097 = local read "upright"() -> (w5222:bool)
                                n2098 = local read "upleft"() -> (w5225:bool)
                                n2099 = local read "down"() -> (w5221:bool)
                                n2100 = local read "right"() -> (w5223:bool)
                                n2101 = local read "left"() -> (w5219:bool)
                                n2102 = local read "up"() -> (w5224:bool)
                                n2103 = call "movestageparams.vi"("command"="get") -> ("Params out"=w5228:T20)  [unwired: 1 in]
                                n2104 = Bundle By Name(cluster=w5228, "upleft"=w5225, "up"=w5224, "upright"=w5222, "right"=w5223, "downright"=w5218, "down"=w5221, "downleft"=w5220, "left"=w5219, "Bigsmall"=w5217) -> (w5229:T20)
                                n2105 = call "movestageparams.vi"("Params in"=w5229, "command"="set") -> ()  [unwired: 1 out]
                                }
                                frame #1 {
                                n2106 = call "movestage.vi"() -> ()  [unwired: 12 in]
                                }
                                frame #2 {
                                w5230 = FALSE ("OK Button")
                                w5231 = FALSE ("OK Button")
                                n2107 = property on="down" class="Bool (strict)"("Value"=w5231) -> ()  [unwired: 2 in, 2 out]
                                n2108 = property on="up" class="Bool (strict)"("Value"=w5231) -> ()  [unwired: 2 in, 2 out]
                                n2109 = property on="right" class="Bool (strict)"("Value"=w5231) -> ()  [unwired: 2 in, 2 out]
                                n2110 = property on="left" class="Bool (strict)"("Value"=w5231) -> ()  [unwired: 2 in, 2 out]
                                n2111 = property on="upleft" class="Bool (strict)"("Value"=w5230) -> ()  [unwired: 2 in, 2 out]
                                n2112 = property on="upright" class="Bool (strict)"("Value"=w5230) -> ()  [unwired: 2 in, 2 out]
                                n2113 = property on="downleft" class="Bool (strict)"("Value"=w5230) -> ()  [unwired: 2 in, 2 out]
                                n2114 = property on="downright" class="Bool (strict)"("Value"=w5230) -> ()  [unwired: 2 in, 2 out]
                                }
                                }
                                }
                                }
                                }
                              }
                              n2115 = dll-call lib="phlib.dll" fn="_PH_GetCountRate@8" label="PH_GetCountRate"("devidx"=w5177, "channel"=1) -> (→"Ch1Rate":i32)  [unwired: 5 in, 2 out]
                              n2116 = local read "Stop"() -> (w5179:bool)
                              n2117 = local write "points recorded"(w5176) -> ()
                            }
                          }
                          frame #3 {
                            w5239 = FALSE ("Value (Signaling)")
                            n2118 = call "2pparameters.vi"("command"="get") -> ("params out"=w5233:T10)  [unwired: 1 in]
                            n2119 = Unbundle By Name(w5233) -> ("autoshutter"=w5234:bool)
                            n2120 = case shown="True" w5234 {
                              frame False {
                              }
                              frame True {
                                n2121 = call "shuttercontrol.vi"("command"="close") -> ()  [unwired: 1 in, 1 out]
